vi "New.vi"(0 "Topic":string, 5 "Arguments Payload":string="[]", 7 "ArgumentKw Payload":string="{}", 9 "Details":string="[]", 11 "ErrorOrSuccess JSON":refnum<class "ErrorOrSuccess JSON.lvclass">) -> (4 "CallResult JSON out":refnum<class "CallResult JSON.lvclass">)   [LabVIEW 2020, in "wamplv.lvlib" / "CallResult JSON.lvclass"]
uses:
  CallResult JSON.lvclass
  CallResult JSON.lvclass/CallResult JSON.ctl
  Message loop classes/ErrorOrSuccess JSON/ErrorOrSuccess JSON.lvclass
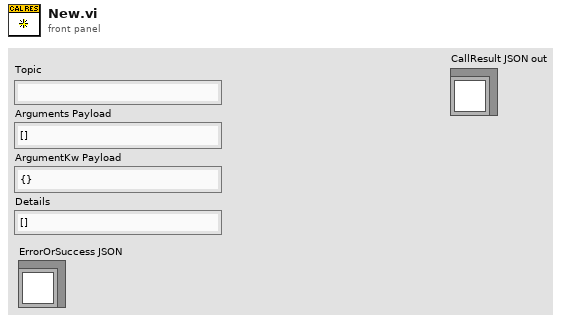
[diagram p1: front panel]
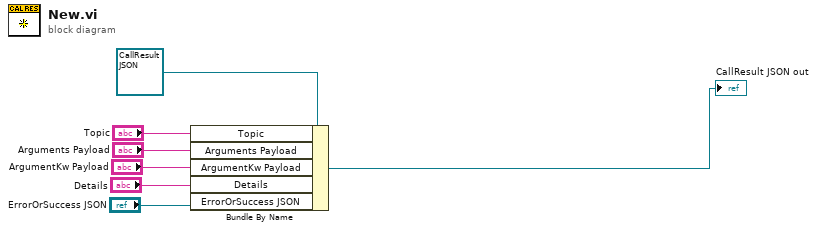
[diagram p0: block diagram]
diagram:
  n1 = Bundle By Name(cluster=refnum<class "CallResult JSON.lvclass"> refnum ("wamplv.lvlib:CallResult JSON.lvclass"), "Topic"="Topic", "Arguments Payload"="Arguments Payload", "ArgumentKw Payload"="ArgumentKw Payload", "Details"="Details", "ErrorOrSuccess JSON"="ErrorOrSuccess JSON") -> (→"CallResult JSON out":refnum<class "CallResult JSON.lvclass">)
